vi "Initialise.vi"(8 "error in (no error)":errorcluster, 11 "Node in":refnum<class "bt_Send_Synch_WithValues.lvclass">) -> (0 "error out":errorcluster, 3 "Node out":refnum<class "bt_Send_Synch_WithValues.lvclass">)   [LabVIEW 2021, in "BT.lvlib" / "bt_Send_Synch_WithValues.lvclass"]
uses:
  bt_Send_Synch_WithValues.lvclass
  bt_Send_Synch_WithValues.lvclass/bt_Send_Synch_WithValues.ctl
  Parent/Send/bt_Send_Synch.lvclass
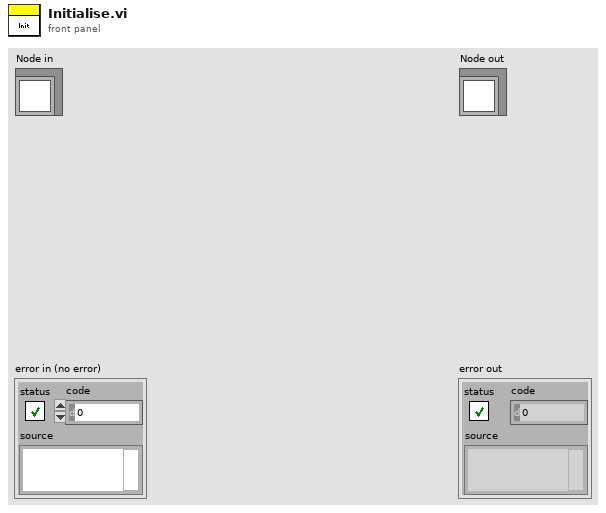
[diagram p1: front panel]
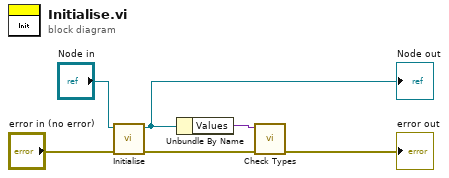
[diagram p0: block diagram]
diagram:
  n1 = call-parent "Initialise.vi"("error in (no error)"="error in (no error)", "Node in"="Node in") -> ("error out"=w4:errorcluster, "Node out"=w3:refnum<class "bt_Send_Synch_WithValues.lvclass">)  [unwired: 8 in]
  "Node out" <- w3
  n2 = Unbundle By Name(w3) -> ("Values"=w2:variant)
  n3 = call "Check Types.vi"("error in (no error)"=w4, "Variant"=w2) -> ("error out"=→"error out":errorcluster)  [unwired: 9 in]
